vi "Periodic Tasks-Periodic Swerve.vi"(8 "error in":errorcluster) -> ()   [LabVIEW 2015]
doc: "This VI runs in parallel to other tasks. It can contain as many user-defined periodic loops as you need. These can carry out PID or other sorts of timed response."
uses:
  Robot Global Data.vi
panel:
  out "Z axis":dbl
  out "Y  axis":dbl
  out "X axis":dbl
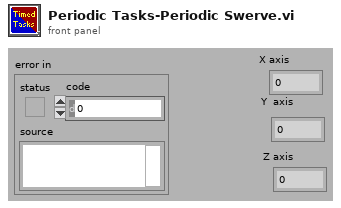
[diagram p1: front panel]
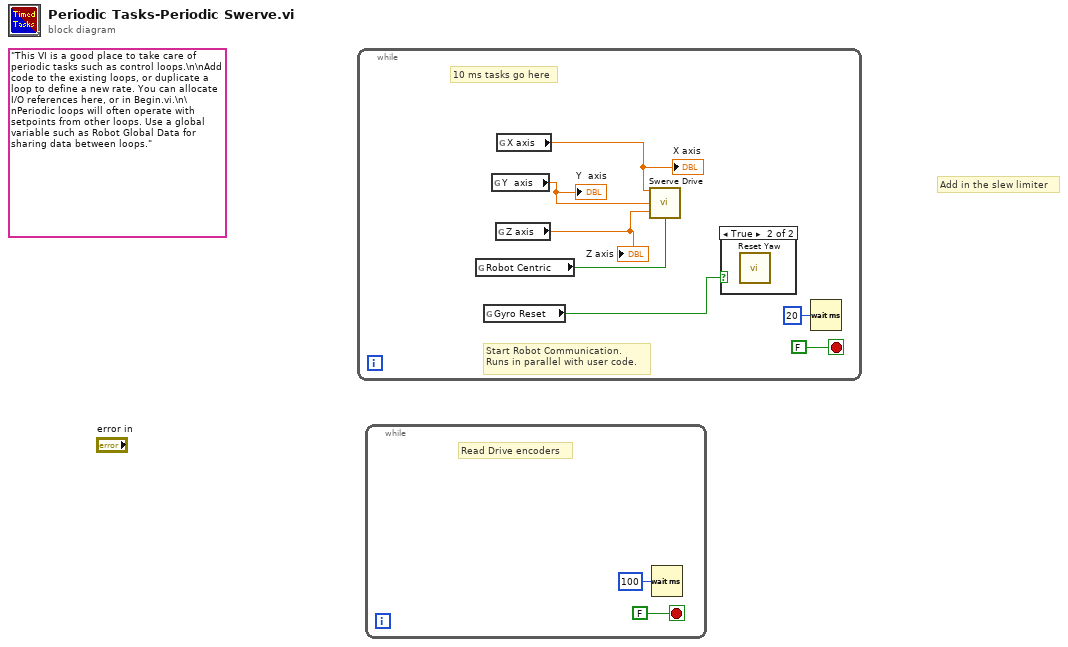
[diagram p0: block diagram]
diagram:
  (unwired) "This VI is a good place to take care of periodic tasks such as control loops.\n\nAdd code to the existing loops, or duplicate a loop to define a new rate. You can allocate I/O references here, or in Begin.vi.\n\nPeriodic loops will often operate with setpoints from other loops. Use a global variable such as Robot Global Data for sharing data between loops."
  # "Add in the slew limiter"
  n1 = while {
    stop <- FALSE stop-if-true
    # "Start Robot Communication.\nRuns in parallel with user code."
    # "10 ms tasks go here"
    n2 = global read "Robot Global Data.vi" "Robot Centric"() -> (w3:bool)
    n3 = global read "Robot Global Data.vi" "Gyro Reset"() -> (w4:bool)
    n4 = global read "Robot Global Data.vi" "Y  axis"() -> (w2:dbl)
    "Y  axis" <- w2
    n5 = global read "Robot Global Data.vi" "Z axis"() -> (w5:dbl)
    "Z axis" <- w5
    n6 = global read "Robot Global Data.vi" "X axis"() -> (w1:dbl)
    "X axis" <- w1
    n7 = call "Swerve Drive.vi"("X"=w1, "Y"=w2, "Z"=w5, "Robot-Centric"=w3) -> ()  [unwired: 12 in]
    n8 = case shown="True" w4 {
      frame False {
      }
      frame True {
        n9 = call "Reset Yaw.vi"() -> ()  [unwired: 12 in]
      }
    }
    n10 = Wait (ms)(milliseconds to wait=u32 20) -> ()  [unwired: 1 out]
  }
  n11 = while {
    stop <- FALSE stop-if-true
    # "Read Drive encoders"
    n12 = Wait (ms)(milliseconds to wait=u32 100) -> ()  [unwired: 1 out]
  }
